vi "Access example.vi"() -> ()   [LabVIEW 2016]
uses:
  Access/Access Lib.lvlib
panel:
  out "error out":errorcluster
  in  "error in (no error)":errorcluster
  in  "是否创建唯一键":bool
  in  "columns":T1={"时间"=timestamp(3701329794.75653 s since 1904-01-01), "测量模式"="水样测试", "数据类型"="N", "检测值"=0.0, "单位"="mg/L", "数据标识"="N", "X"=0.0, "量程标识"="", "SN"="", "标样参考值"=0.0, "跨度值"=0.0, "F0"=0.0, "F1"=0.0, "F2"=0.0, "F3"=0.0, "F4"=0.0, "F5"=0.0, "F6"=0.0, "F7"=0.0, "X1"=0.0, "因子编码"="", "温度"=0.0, "湿度"=0.0, "测量量程"=0.0, "测量检出限"=0.0, "测量精度"=0.0, "测量间隔"=0.0, "消解温度"=0.0, "消解时长"=0.0, "三项式系数"=0.0, "二次多项式系数"=0.0, "曲线斜率"=0.0, "曲线截距"=0.0, "线性相关系数"=0.0, "空白校准时间"=timestamp(0 s since 1904-01-01), "标样校准时间"=timestamp(0 s since 1904-01-01), "测量信号值"=0.0, "稀释倍数"=0.0, "空白标定系数"=0.0, "量程系数"=0.0, "LastTime"=timestamp(0 s since 1904-01-01)}
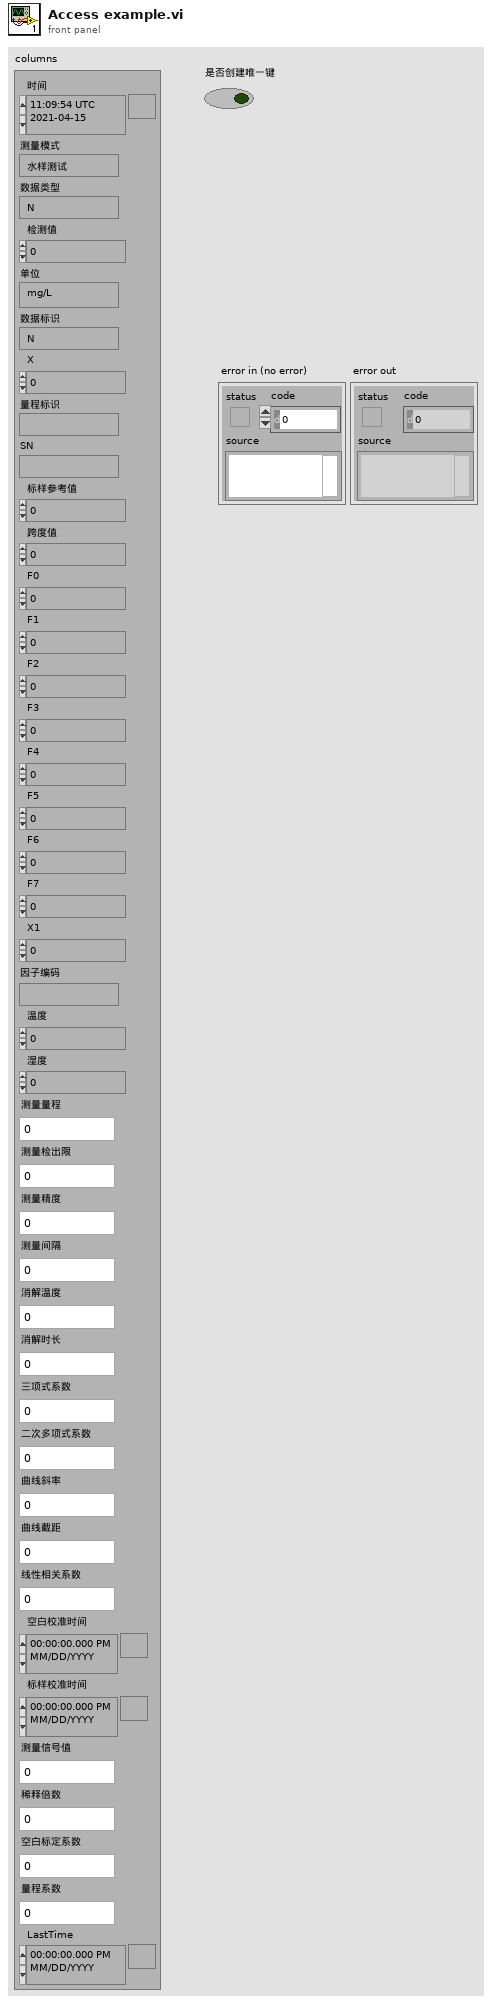
[diagram p1: front panel]
types:
  T1 = typedef "营养盐字段定义.ctl" = cluster{"时间":timestamp, "测量模式":string, "数据类型":string, "检测值":sgl, "单位":string, "数据标识":string, "X":sgl, "量程标识":string, "SN":string, "标样参考值":sgl, "跨度值":sgl, "F0":sgl, "F1":sgl, "F2":sgl, "F3":sgl, "F4":sgl, "F5":sgl, "F6":sgl, "F7":sgl, "X1":sgl, "因子编码":string, "温度":sgl, "湿度":sgl, "测量量程":sgl, "测量检出限":sgl, "测量精度":sgl, "测量间隔":sgl, "消解温度":sgl, "消解时长":sgl, "三项式系数":sgl, "二次多项式系数":sgl, "曲线斜率":sgl, "曲线截距":sgl, "线性相关系数":sgl, "空白校准时间":timestamp, "标样校准时间":timestamp, "测量信号值":sgl, "稀释倍数":sgl, "空白标定系数":sgl, "量程系数":sgl, "LastTime":timestamp}
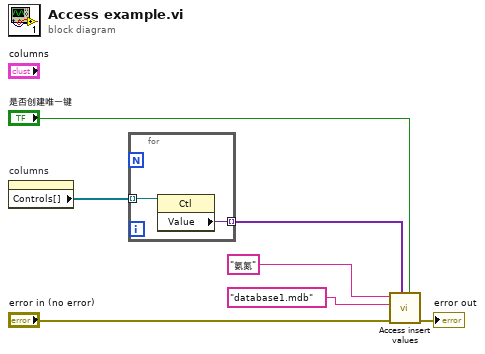
[diagram p0: block diagram]
diagram:
  n1 = property on="columns" class="Clust (严格)"() -> ("Controls[]"=w6:refnum<vi>[])  [unwired: 2 in, 2 out]
  n2 = for {
    tunnel: w6 -> [w9] mode=indexing
    tunnel: [w8] -> w5 mode=indexing
    n3 = property class="Ctl"(reference=w9) -> ("Value"=w8:variant)  [unwired: 1 in, 2 out]
  }
  n4 = call "Access insert values.vi"("是否创建唯一键"="是否创建唯一键", "data"=w5, "error in (no error)"="error in (no error)", "database"="database1.mdb", "table"="氨氮") -> ("error out"=→"error out":errorcluster)  [unwired: 6 in]
